vi "zad3.vi"() -> ()   [LabVIEW 2017]
uses:
  <vilib>/sound2/lvsound2.llb/Sound File Read Open.vi
  <vilib>/sound2/lvsound2.llb/Sound File Read (DBL).vi
panel:
  in  "stop":bool
  in  "path":path
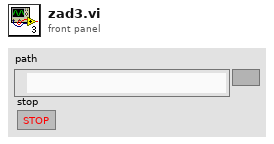
[diagram p1: front panel]
types:
  T1 = typedef "Sound File Refnum.ctl" = refnum<file>
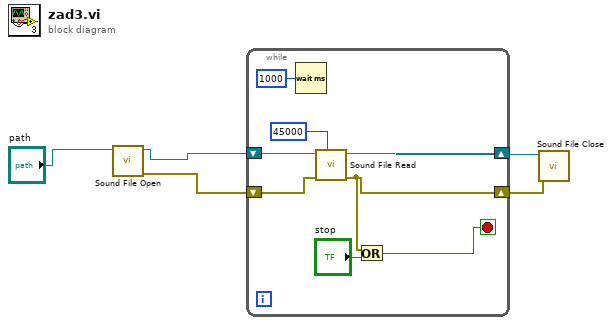
[diagram p0: block diagram]
diagram:
  n1 = call-poly <vilib>:"Sound File Open.vi"("path"="path") -> ("error out"=w1:errorcluster, "sound file refnum"=w2:T1)  [unwired: 9 in]
  n2 = while {
    shift-right: [w9] -> w5
    shift-left: w1 -> [w13]
    shift-right: [w10] -> w4
    shift-left: w2 -> [w12]
    stop <- w7 stop-if-true
    n3 = Wait (ms)(milliseconds to wait=u32 1000) -> ()  [unwired: 1 out]
    n4 = call-poly <vilib>:"Sound File Read.vi"("number of samples/ch (-1: all)"=45000, "error in (no error)"=w13, "sound file refnum"=w12) -> ("error out"=w9:errorcluster, "sound file refnum out"=w10:T1)  [unwired: 4 in, 3 out]
    n5 = Or(x=w9, y="stop") -> (x .or. y?=w7:bool)
  }
  n6 = call <vilib>:"Sound File Close.vi"("error in (no error)"=w5, "sound file refnum"=w4) -> ()  [unwired: 9 in, 1 out]
